vi "OPCUA Initialzie.vi"(6 "SUbscription Node IDs":string, 7 "publishing interval (10 ms)":dbl=10.0 format="%#_13g", 8 "error in (no error)":errorcluster, 10 "OPCUA Initialize":bool, 11 "Model_AMC in":refnum<class "Model_AMC.lvclass">) -> (0 "error out":errorcluster, 2 "OPCUA Even":T1, 3 "Model_AMC out":refnum<class "Model_AMC.lvclass">)   [LabVIEW 2021, in "Model_AMC.lvclass"]
uses:
  Model_AMC.lvclass
  Model_AMC.lvclass/Model_AMC.ctl
  <userlib>/John_Lib/OPCUA/OPCUA.lvclass
  <vilib>/OPCUA/controls/Subscription ID.ctl
  <vilib>/OPCUA/controls/OPC UA StatusCode.ctl
  <vilib>/OPCUA/controls/Data Type.ctl
  <vilib>/OPCUA/controls/NodeId.ctl
  <vilib>/OPCUA/controls/Subscription Data Change.ctl
  <userlib>/John_Lib/OPCUA/ReSubscription Even.ctl
  <userlib>/John_Lib/OPCUA/OPCUA Even.ctl
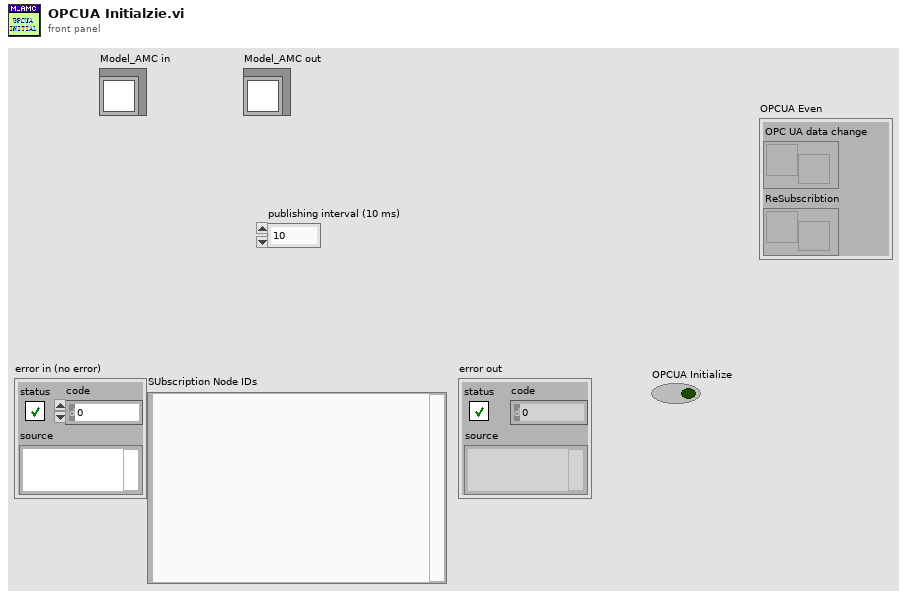
[diagram p1: front panel]
types:
  T1 = typedef "OPCUA.lvlib/OPCUA.lvclass/OPCUA Even.ctl" = cluster{"OPC UA data change":refnum<user-event>, "ReSubscribtion":refnum<user-event>}
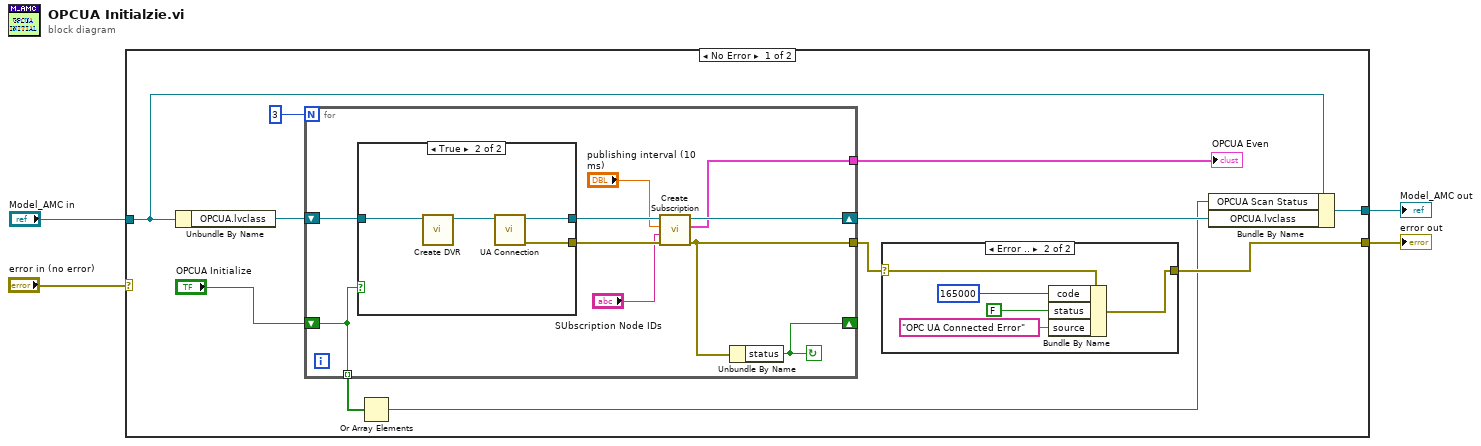
[diagram p0: block diagram]
diagram:
  n1 = case shown="No Error" "error in (no error)" {
    selector: "error in (no error)" -> [_ w37]
    tunnel: [w8 w37] -> w4
    tunnel: [w12 w38] -> w1
    tunnel: "Model_AMC in" -> [w11 w38]
    frame No Error {
      n2 = Unbundle By Name(w11) -> ("OPCUA.lvclass"=w13:refnum<class "OPCUA.lvclass">)
      n3 = for {
        N: 3 -> [_]
        tunnel: [w29] -> w14
        tunnel: [w22] -> w9
        shift-right: [w30] -> w15
        shift-left: w13 -> [w28]
        shift-right: [w26] -> _
        shift-left: "OPCUA Initialize" -> [w25]
        tunnel: [w25] -> w7 mode=indexing
        stop <- w26 continue-if-true
        n4 = case shown="True" w25 {
          tunnel: [w32 w36] -> w31
          tunnel: w28 -> [w32 w35]
          tunnel: [_ w33] -> w27
          frame False {
          }
          frame True {
            n5 = call <userlib>:"Create DVR.vi"("OPCUA in"=w35) -> ("OPCUA out"=w34:refnum<class "OPCUA.lvclass">)  [unwired: 9 in, 1 out]
            n6 = call <userlib>:"UA Connection.vi"("OPCUA in"=w34) -> ("error out"=w33:errorcluster, "OPCUA out"=w36:refnum<class "OPCUA.lvclass">)  [unwired: 9 in]
          }
        }
        n7 = call <userlib>:"Create Subscription.vi"("error in (no error)"=w27, "Node IDs"="SUbscription Node IDs", "publishing interval (10 ms)"="publishing interval (10 ms)", "OPCUA in"=w31) -> ("error out"=w22:errorcluster, "Even"=w29:T1, "OPCUA out"=w30:refnum<class "OPCUA.lvclass">)  [unwired: 5 in]
        n8 = Unbundle By Name(w22) -> ("status"=w26:bool)
      }
      "OPCUA Even" <- w14
      n9 = Or Array Elements(Boolean array=w7) -> (logical OR=w5:bool)
      n10 = case shown="Error .." w9 {
        selector: w9 -> [w16 w19]
        tunnel: [w16 w17] -> w8
        frame No Error {
        }
        frame Error {
          n11 = Bundle By Name(cluster=w19, "code"=165000, "status"=FALSE, "source"="OPC UA Connected Error") -> (w17:errorcluster)
        }
      }
      n12 = Bundle By Name(cluster=w11, "OPCUA Scan Status"=w5, "OPCUA.lvclass"=w15) -> (w12:refnum<class "Model_AMC.lvclass">)
    }
    frame Error {
    }
  }
  "error out" <- w4
  "Model_AMC out" <- w1
